vi "Part 7 Build Matrix.vi"() -> ()   [LabVIEW 2020]
uses:
  <vilib>/Analysis/Matrix/Datatypes/RealMatrix.ctl
  <vilib>/Analysis/Matrix/NI_Matrix.lvlib
panel:
  out "appended array":T1
  in  "element 2":dbl[](array[numeric])
  in  "element":dbl[](array[numeric])
  # "Build Matrix"
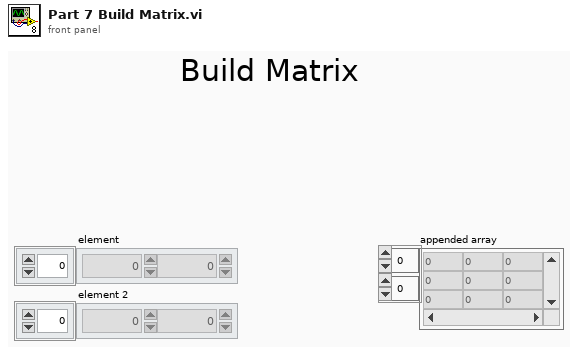
[diagram p1: front panel]
types:
  T1 = typedef "NI_Matrix.lvlib/RealMatrix.ctl" = dbl[][]
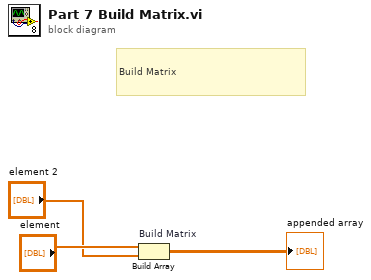
[diagram p0: block diagram]
diagram:
  # "Build Matrix"
  n1 = Build Array "Build Matrix"("element", "element 2") -> (→"appended array":T1)
